vi "DVR Access.vi"(0 "Input":dbl, 2 "Stop":bool, 11 "Error In":errorcluster) -> (4 "Output":dbl, 15 "Error Out":errorcluster)   [LabVIEW 2019]
doc: "This VI creates a DVR and passes it to 4 loops and performs operation in 3 loops and read the data value in the 4th loop."
panel:
  # "Instruction:\n\n1. Run the VI.\n2. Specify the input.\n3. Observe the output in the indicator.\n4. Press stop to stop running the VI.\n5. Open the block diagram and make changes in the wait time, settings of the in place element to observe the behaviour of DVRs."
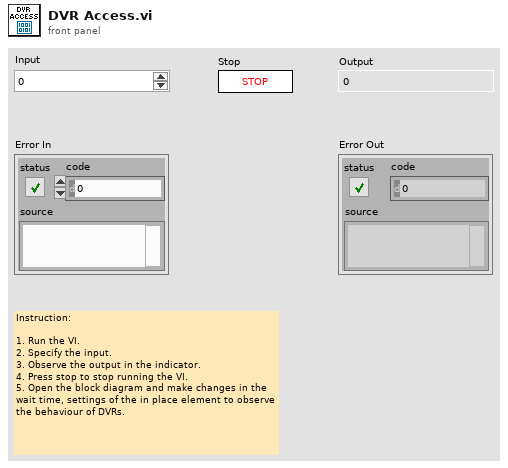
[diagram p1: front panel]
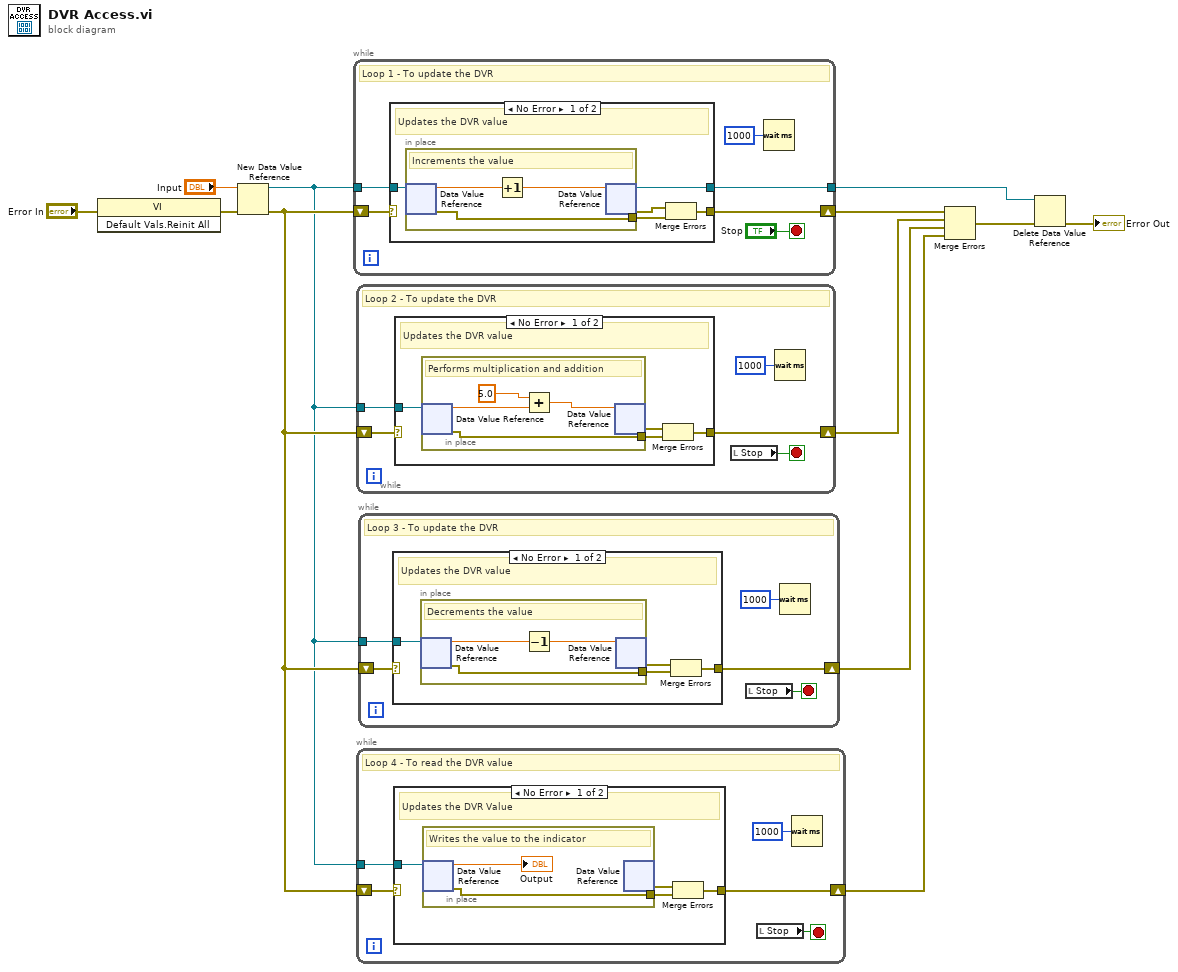
[diagram p0: block diagram]
diagram:
  n1 = invoke class="VI" method="Default Vals.Reinit All"(error in="Error In") -> (error out=w1:errorcluster)  [unwired: 2 in, 2 out]
  n2 = New Data Value Reference(data value="Input", error in=w1) -> (data value reference=w2:refnum<data-value>, error out=w5:errorcluster)
  n3 = while {
    shift-right: [w14] -> w11
    shift-left: w5 -> [w13]
    tunnel: w2 -> [w17]
    tunnel: [w16] -> w6
    stop <- "Stop" stop-if-true
    # "Loop 1 - To update the DVR"
    n4 = case shown="No Error" w13 {
      selector: w13 -> [_ w27]
      tunnel: w17 -> [w23 w28]
      tunnel: [w22 w28] -> w16
      tunnel: [w21 w27] -> w14
      frame No Error {
        # "Updates the DVR value"
        n5 = in-place {
          in-place-border: [w24] -> w19
          # "Increments the value"
          n6 = in-place-dvr #1(w23) -> (w25:dbl, w24:errorcluster)
          n7 = Increment(x=w25) -> (x+1=w26:dbl)
          n8 = in-place-dvr #1(w26) -> (w22:refnum<data-value>, w20:errorcluster)
        }
        n9 = Merge Errors(w20, w19) -> (w21:errorcluster)
      }
      frame Error {
      }
    }
    n10 = Wait (ms)(milliseconds to wait=u32 1000) -> ()  [unwired: 1 out]
  }
  n11 = while {
    shift-right: [w30] -> w3
    shift-left: w5 -> [w29]
    tunnel: w2 -> [w32]
    stop <- w31 stop-if-true
    # "Loop 2 - To update the DVR"
    n12 = case shown="No Error" w29 {
      selector: w29 -> [_ w42]
      tunnel: w32 -> [w37 _]
      tunnel: [w35 w42] -> w30
      frame No Error {
        # "Updates the DVR value"
        n13 = in-place {
          in-place-border: [w38] -> w34
          # "Performs multiplication and addition"
          n14 = in-place-dvr #2(w37) -> (w40:dbl, w38:errorcluster)
          n15 = Add(x=5.0, y=w40) -> (x+y=w39:dbl)
          n16 = in-place-dvr #2(w39) -> (w36:errorcluster)  [unwired: 1 out]
        }
        n17 = Merge Errors(w36, w34) -> (w35:errorcluster)
      }
      frame Error {
      }
    }
    n18 = local read "Stop"() -> (w31:bool)
    n19 = Wait (ms)(milliseconds to wait=u32 1000) -> ()  [unwired: 1 out]
  }
  n20 = while {
    shift-right: [w44] -> w8
    shift-left: w5 -> [w43]
    tunnel: w2 -> [w47]
    stop <- w45 stop-if-true
    # "Loop 4 - To read the DVR value"
    n21 = case shown="No Error" w43 {
      selector: w43 -> [_ w54]
      tunnel: w47 -> [w51 _]
      tunnel: [w48 w54] -> w44
      frame No Error {
        # "Updates the DVR Value"
        n22 = in-place {
          in-place-border: [w53] -> w49
          # "Writes the value to the indicator"
          n23 = in-place-dvr #3(w51) -> (→"Output":dbl, w53:errorcluster)
          n24 = in-place-dvr #3() -> (w50:errorcluster)  [unwired: 1 in, 1 out]
        }
        n25 = Merge Errors(w50, w49) -> (w48:errorcluster)
      }
      frame Error {
      }
    }
    n26 = local read "Stop"() -> (w45:bool)
    n27 = Wait (ms)(milliseconds to wait=u32 1000) -> ()  [unwired: 1 out]
  }
  n28 = while {
    shift-right: [w56] -> w4
    shift-left: w5 -> [w55]
    tunnel: w2 -> [w59]
    stop <- w57 stop-if-true
    # "Loop 3 - To update the DVR"
    n29 = case shown="No Error" w55 {
      selector: w55 -> [_ w67]
      tunnel: w59 -> [w63 _]
      tunnel: [w60 w67] -> w56
      frame No Error {
        # "Updates the DVR value"
        n30 = in-place {
          in-place-border: [w64] -> w61
          # "Decrements the value"
          n31 = in-place-dvr #4(w63) -> (w66:dbl, w64:errorcluster)
          n32 = Decrement(x=w66) -> (x-1=w65:dbl)
          n33 = in-place-dvr #4(w65) -> (w62:errorcluster)  [unwired: 1 out]
        }
        n34 = Merge Errors(w62, w61) -> (w60:errorcluster)
      }
      frame Error {
      }
    }
    n35 = local read "Stop"() -> (w57:bool)
    n36 = Wait (ms)(milliseconds to wait=u32 1000) -> ()  [unwired: 1 out]
  }
  n37 = Merge Errors(w11, w3, w4, w8) -> (w9:errorcluster)
  n38 = Delete Data Value Reference(data value reference=w6, error in=w9) -> (error out=→"Error Out":errorcluster)  [unwired: 1 out]
